vi "GetConstructorInfo.vi"(6 "Style ID":u32, 8 "error in":errorcluster, 11 "PythonConverter_GUI in":refnum<class "PythonConverter_GUI.lvclass">) -> (0 "error out":errorcluster, 2 "found":bool, 3 "PythonConverter_GUI out":refnum<class "PythonConverter_GUI.lvclass">, 4 "Constructor Info":T1)   [LabVIEW 2014, in "PythonConverter_GUI.lvclass"]
uses:
  PythonConverter_GUI.lvclass
  TypeDefs/ConstructorInfo.ctl
  PythonConverter_GUI.lvclass/PythonConverter_GUI.ctl
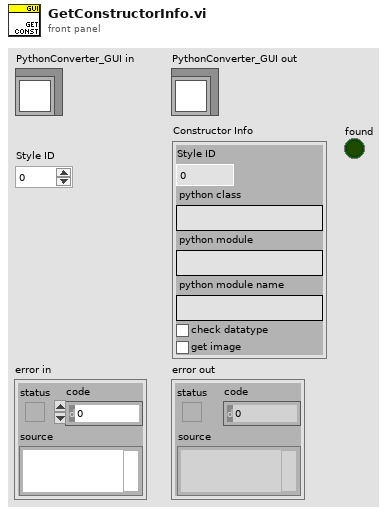
[diagram p1: front panel]
types:
  T1 = typedef "PythonConverter_GUI.lvclass/ConstructorInfo.ctl" = cluster{"Style ID":u32, "python class":string, "python module":string, "python module name":string, "check datatype":bool, "get image":bool}
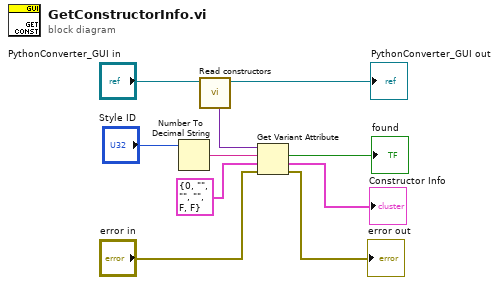
[diagram p0: block diagram]
diagram:
  n1 = Number To Decimal String(number="Style ID") -> (decimal integer string=w7:string)  [unwired: 1 in]
  n2 = call "Read constructors.vi"("PythonConverter_GUI in"="PythonConverter_GUI in") -> ("PythonConverter_GUI out"=→"PythonConverter_GUI out":refnum<class "PythonConverter_GUI.lvclass">, "constructors"=w8:variant)  [unwired: 7 in]
  n3 = Get Variant Attribute(Variant=w8, name=w7, default value (empty Variant)=T1 {"Style ID"=0, "python class"="", "python module"="", "python module name"="", "check datatype"=FALSE, "get image"=FALSE} ("Constructor Info"), error in="error in") -> (found=→"found":bool, value=→"Constructor Info":T1, error out=→"error out":errorcluster)  [unwired: 1 out]
